vi "HEX String Decode.vi"(8 "Values To Decode":u16, 10 "String In":string) -> (1 "Array":u32[](array[numeric]) format="%x", 3 "Remaining String":string)   [LabVIEW 2014]
panel:
  # "Decode some or all of a HEX string to HEX values"
  # "To decode entire string,\nset Values To Decode = 0"
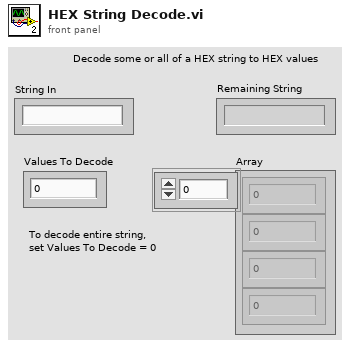
[diagram p1: front panel]
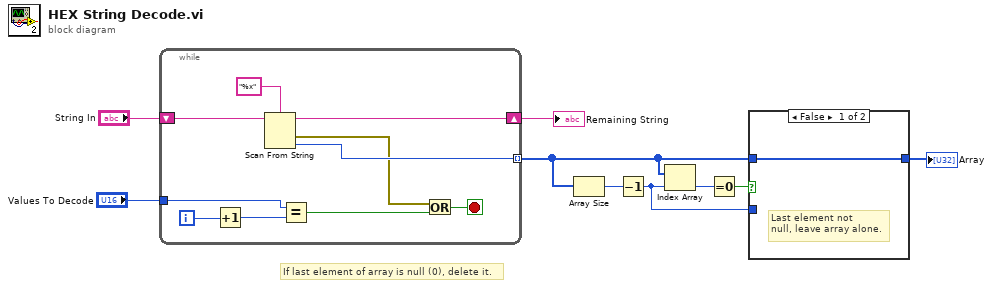
[diagram p0: block diagram]
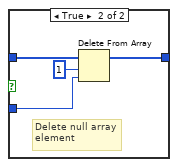
[diagram p2: hidden frame]
diagram:
  # "If last element of array is null (0), delete it."
  n1 = while {
    shift-right: [w17] -> w8
    shift-left: "String In" -> [w18]
    tunnel: [w16] -> w3 mode=indexing
    tunnel: "Values To Decode" -> [w11]
    i -> [w13]
    stop <- w14 stop-if-true
    n2 = Increment(x=w13) -> (x+1=w12:i32)
    n3 = Scan From String "Scan From String"(format string="%x", input string=w18) -> (remaining string=w17:string, error out=w15:errorcluster, output 1=w16:u32)  [unwired: 3 in, 1 out]
    n4 = Equal?(x=w11, y=w12) -> (x = y?=w10:bool)
    n5 = Or(x=w15, y=w10) -> (x .or. y?=w14:bool)
  }
  "Remaining String" <- w8
  n6 = Array Size(array=w3) -> (size(s)=w6:i32)
  n7 = Decrement(x=w6) -> (x-1=w2:i32)
  n8 = Index Array(array=w3, index=w2) -> (element=w5:u32)
  n9 = Equal To 0?(x=w5) -> (x = 0?=w4:bool)
  n10 = case shown="False" w4 {
    tunnel: w3 -> [w20 w24]
    tunnel: w2 -> [_ w22]
    tunnel: [w20 w21] -> w1
    frame False {
      # "Last element not\nnull, leave array alone."
    }
    frame True {
      # "Delete null array\nelement"
      n11 = Delete From Array(array=w24, length=1, index=w22) -> (array with subset deleted=w21:u32[])  [unwired: 1 out]
    }
  }
  "Array" <- w1
